vi "Servo_init.vi"(2 "error in (no error)":errorcluster) -> (0 "error out":errorcluster)   [LabVIEW 2009, in "Servo.lvlib"]
doc: "This is the initialisation function for the servos used on the robot. The function has a few different purposes. \n\nThe function reads the ServoSettings.ini and stores all the configuration inside the variable Servo_Config. This file contains information about what pulse (with a period of 20,000 uSec) that represent the middle position, the 45deg to right position, the 45deg to left position for some servo. This is for calibration purposes. If more servos than the original ones are added an entry for that particular servo will need to be added inside the ServoSettings.ini\n\nThe function also enables the sending of PWM signals to PWM9 and PWM10, this also will need to be changed if more servos are added.\n\nWhen Servo_init is run PWM9 and PWM10 will be set to their initial position in 0deg. This value will then be stored in the variable Servo_Angles that keeps track of where the servos are at that time.\n\nThe function only needs to be called once in the beginning. But it will need to be have a reference to the FPGA to work."
uses:
  Servo.lvlib
  PWM/PWM_Name.ctl
  <vilib>/Utility/config.llb/Read Key (Double).vi
  <vilib>/Utility/config.llb/NI_LVConfig.lvlib
  PWM.lvlib
  Utility.lvlib
panel:
  out "String":string
  out "appended array 2":string[](array[string])
  in  "error in (no error) 2":errorcluster
  out "Array 2":T1(array[cluster])
  out "appended array":string[](array[string])
  out "appended path":path
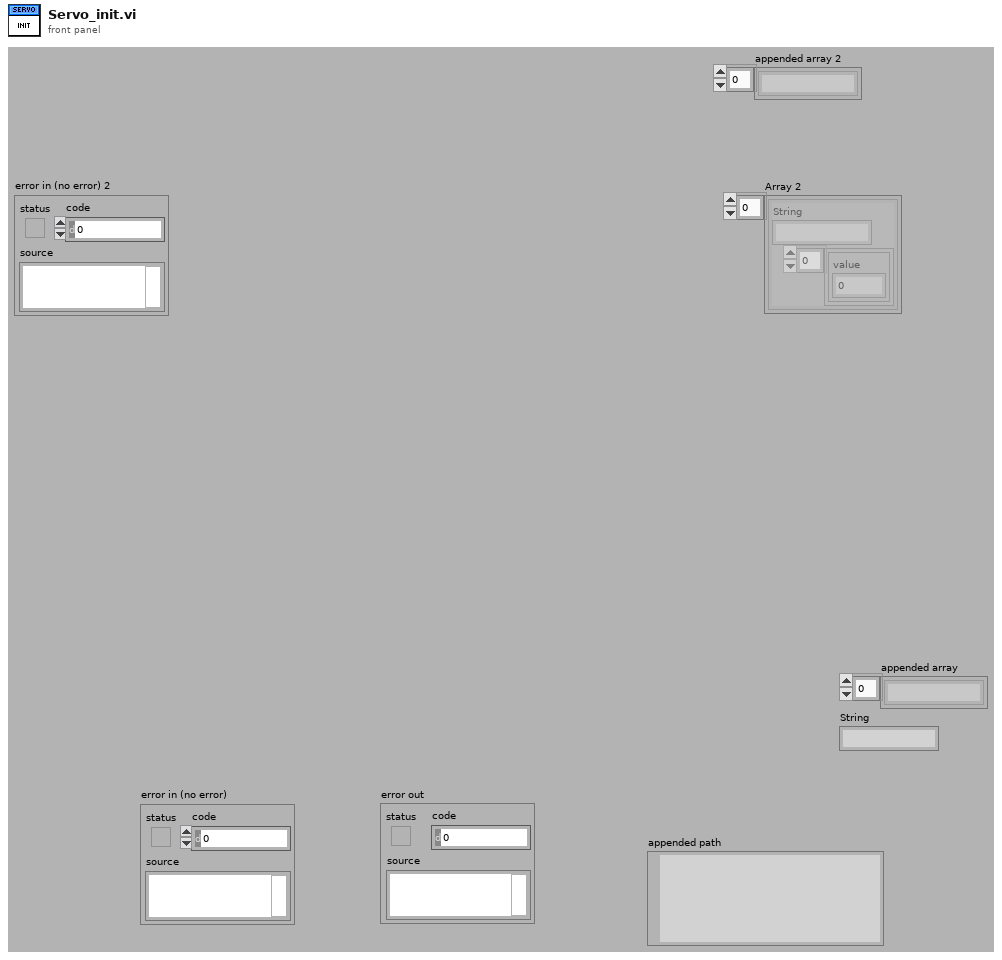
[diagram p1: front panel]
types:
  T1 = cluster{"String":string, cluster{"value":dbl}[]}[]
  T2 = typedef "PWM.lvlib/PWM_Name.ctl" = u16
  T3 = typedef "NI_LVConfig.lvlib/Config Data RefNum.ctl" = refnum<k1>
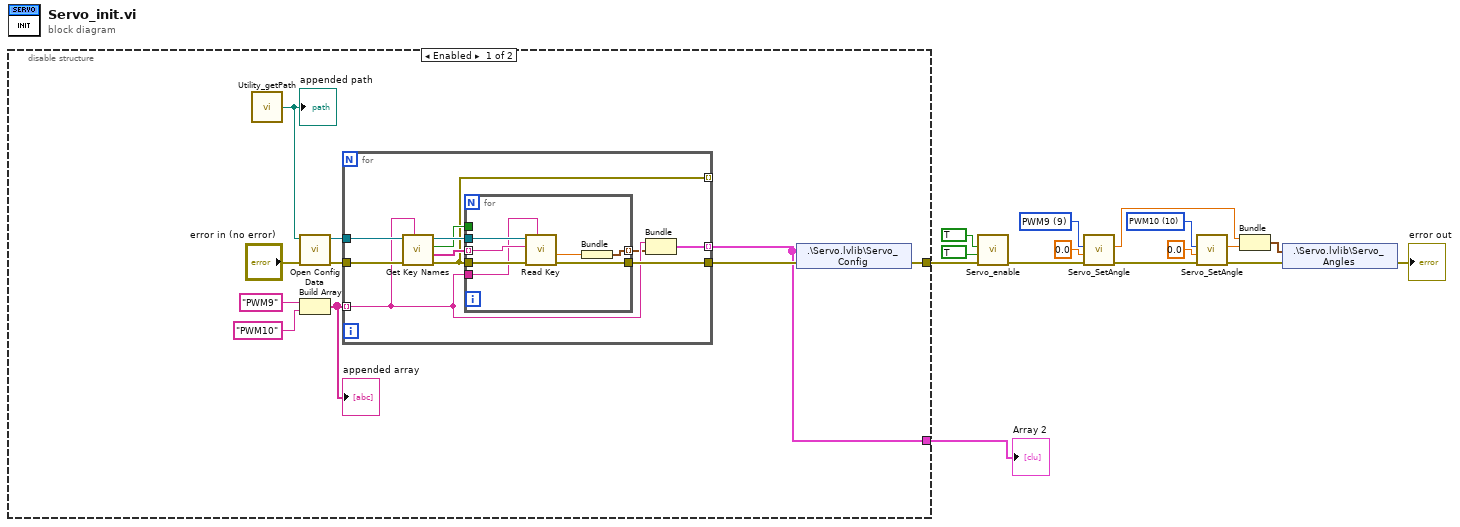
[diagram p0: block diagram]
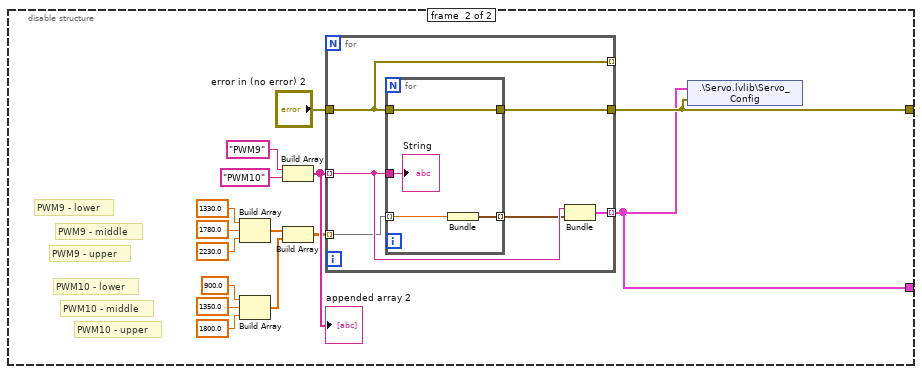
[diagram p2: hidden frame]
diagram:
  w10 = T2 9 items=["Invalid"=0, "PWM1"=1, "PWM2"=2, "PWM9"=9, "PWM10"=10] ("PWM")
  w11 = T2 10 items=["Invalid"=0, "PWM1"=1, "PWM2"=2, "PWM9"=9, "PWM10"=10] ("PWM")
  n1 = disable-structure shown="Enabled" {
    disable-tunnel: [w23 w54] -> w13
    disable-tunnel: [w16 w43] -> w1
    frame #0 {
      n2 = call "Utility_getPath.vi"() -> ("appended path"=w22:path)  [unwired: 5 in]
      "appended path" <- w22
      n3 = call <vilib>:"Open Config Data.vi"("error in (no error)"="error in (no error)", "configuration file path"=w22) -> ("error out"=w18:errorcluster, "refnum"=w17:T3)  [unwired: 7 in, 1 out]
      n4 = Build Array("PWM9", "PWM10") -> (w19:string[])
      "appended array" <- w19
      n5 = for {
        tunnel: w19 -> [w29] mode=indexing
        tunnel: w17 -> [w32]
        tunnel: w18 -> [w31]
        tunnel: [w30] -> w25
        tunnel: [w28] -> w16 mode=indexing
        tunnel: [w26] -> _ mode=indexing
        n6 = call <vilib>:"Get Key Names.vi"("section"=w29, "error in (no error)"=w31, "refnum"=w32) -> ("error out"=w26:errorcluster, "key names"=w35:string[], "section exists?"=w33:bool, "refnum out"=w34:T3)  [unwired: 5 in]
        n7 = for {
          tunnel: w35 -> [w39] mode=indexing
          tunnel: w26 -> [w42]
          tunnel: w34 -> [w41]
          tunnel: [w40] -> w30
          tunnel: w33 -> [_]
          tunnel: w29 -> [w38]
          tunnel: [w36] -> w27 mode=indexing
          n8 = call-poly <vilib>:"Read Key.vi"("section"=w38, "error in (no error)"=w42, "key"=w39, "refnum"=w41) -> ("error out"=w40:errorcluster, "value"=w37:dbl)  [unwired: 4 in, 2 out]
          n9 = Bundle("value"=w37) -> (w36:cluster{"value":dbl})  [unwired: 1 in]
        }
        n10 = Bundle(w29, w27) -> (w28:cluster{string, cluster{"value":dbl}[]})  [unwired: 1 in]
      }
      n11 = shared-variable ".\\Servo.lvlib\\Servo_Config"(w16, error in=w25) -> (error out=w23:errorcluster)
    }
    frame #1 {
      # "PWM10 - upper"
      # "PWM10 - middle"
      # "PWM10 - lower"
      # "PWM9 - upper"
      # "PWM9 - middle"
      # "PWM9 - lower"
      n12 = Build Array(1330.0 ("Angle in"), 1780.0 ("element"), 2230.0 ("element")) -> (w51:dbl[])
      n13 = Build Array(900.0 ("Angle in"), 1350.0 ("element"), 1800.0 ("element")) -> (w52:dbl[])
      n14 = Build Array("PWM9", "PWM10") -> (w55:string[])
      "appended array 2" <- w55
      n15 = Build Array(w51, w52) -> (w44:dbl[][])
      n16 = for {
        tunnel: w55 -> [w62] mode=indexing
        tunnel: "error in (no error) 2" -> [w59]
        tunnel: [w63] -> w54
        tunnel: [w61] -> w43 mode=indexing
        tunnel: [w59] -> _ mode=indexing
        tunnel: w44 -> [w58] mode=indexing
        n17 = for {
          tunnel: w59 -> [w66]
          tunnel: [w66] -> w63
          tunnel: w62 -> [w64]
          tunnel: [w67] -> w60 mode=indexing
          tunnel: w58 -> [w65] mode=indexing
          n18 = Bundle("element"=w65) -> (w67:cluster{"element":dbl})  [unwired: 1 in]
          "String" <- w64
        }
        n19 = Bundle(w62, w60) -> (w61:cluster{string, cluster{"element":dbl}[]})  [unwired: 1 in]
      }
      n20 = shared-variable ".\\Servo.lvlib\\Servo_Config"(w43, error in=w54) -> ()  [unwired: 1 out]
    }
  }
  "Array 2" <- w1
  n21 = call "Servo_enable.vi"("error in"=w13, "Set PWM9"=TRUE ("Enable 2"), "Set PWM10"=TRUE ("Enable")) -> ("error out"=w9:errorcluster)  [unwired: 8 in]
  n22 = call "Servo_SetAngle.vi"("error in"=w9, "Angle in"=0.0, "PWM"=w10) -> ("error out"=w12:errorcluster, "Angle out"=w5:dbl)  [unwired: 7 in]
  n23 = call "Servo_SetAngle.vi"("error in"=w12, "Angle in"=0.0, "PWM"=w11) -> ("error out"=w3:errorcluster, "Angle out"=w6:dbl)  [unwired: 7 in]
  n24 = Bundle("Angle out"=w5, "Angle out"=w6) -> (w4:cluster{"Angle out":dbl, "Angle out":dbl})  [unwired: 1 in]
  n25 = shared-variable ".\\Servo.lvlib\\Servo_Angles"(w4, error in=w3) -> (error out=→"error out":errorcluster)
